vi "SetParametrPoly.vi"   [LabVIEW 2010, in "StepMotor.lvclass"]
uses:
  StepMotor.lvclass
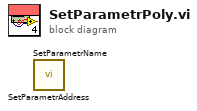
[diagram p0: block diagram]
diagram:
  n1 = call "SetParametrAddress.vi"() -> ()  [unwired: 10 in, 2 out]
  n2 = call "SetParametrName.vi"() -> ()  [unwired: 10 in, 2 out]
